vi "Threshold Detector.vi"(3 "width":i32=1, 4 "threshold":dbl format="%0.2f", 5 "X":dbl[](array[numeric])) -> (0 "error":i32, 1 "count":i32, 2 "Indices":i32[](array[numeric]))   [LabVIEW 2020, in "NI_AALPro.lvlib"]
doc: "Analyzes the input sequence <B>X</B> for valid peaks and keeps a <B>count</B> of the number of peaks encountered and a record of <B>Indices</B>, which locates the points that exceed the <B>threshold</B> in a valid peak."
uses:
  <vilib>/Analysis/NI_AALPro.lvlib
  <resource>/lvanlys.dll
panel:
  # "Threshold Detector"
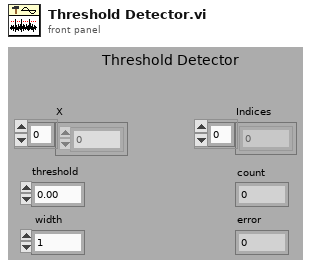
[diagram p1: front panel]
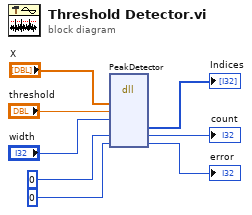
[diagram p0: block diagram]
diagram:
  n1 = dll-call lib="e:/builds/penguin/labview/branches/2020/dev/dist/resource/lvanlys.*" fn="PeakDetector"("X"="X", "threshold"="threshold", "width"="width", 0, 0) -> ("Indices"=→"Indices":i32[], →"count":i32, →"error":i32)  [unwired: 8 in, 2 out]
